vi "GCore_MFP3D_Lucy.vi"(4 "G data":dbl[](array[numeric])=[-0.02172177734863929, 0.0012861831973395592] format="%0.2f", 5 "Femto Gain (V/A)":dbl format="%#_13g", 6 "SR830 sensitivity":dbl=0.1 format="%#_6p", 7 "SR7265 sensitivity (V)":dbl=5e-07 format="%#_6p", 8 "Excitation voltage (V)":dbl format="%#_13g") -> (0 "4tR":dbl format="%#_6p", 1 "4tG":dbl format="%#_6p", 2 "2tR":dbl format="%#_6p", 3 "2tG":dbl format="%#_6p")   [LabVIEW 2019]
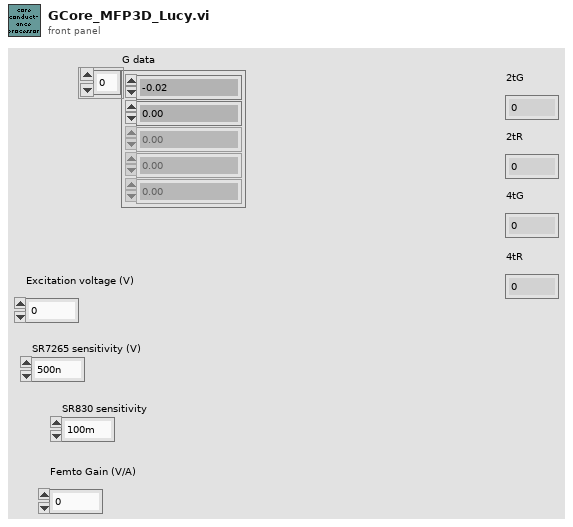
[diagram p1: front panel]
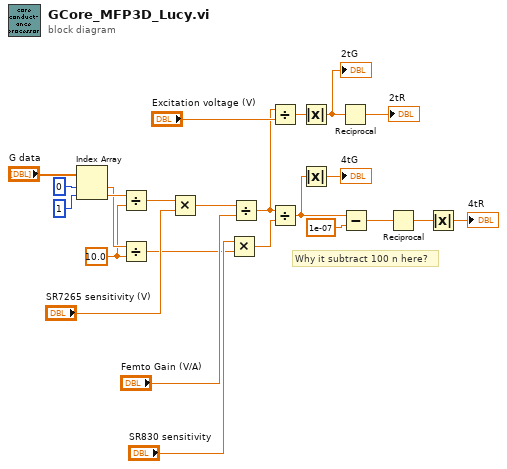
[diagram p0: block diagram]
diagram:
  w14 = 10.0 ("y")
  # "Why it subtract 100 n here?"
  n1 = Index Array(array="G data", index #1=0 ("index"), index #2=1 ("index")) -> (element #1=w15:dbl, element #2=w16:dbl)
  n2 = Divide(x=w16, y=w14) -> (x/y=w19:dbl)
  n3 = Divide(x=w15, y=w14) -> (x/y=w13:dbl)
  n4 = Multiply(x=w19, y="SR7265 sensitivity (V)") -> (x*y=w18:dbl)
  n5 = Multiply(x="SR830 sensitivity", y=w13) -> (x*y=w12:dbl)
  n6 = Divide(x=w18, y="Femto Gain (V/A)") -> (x/y=w11:dbl)
  n7 = Divide(x=w11, y="Excitation voltage (V)") -> (x/y=w10:dbl)
  n8 = Divide(x=w11, y=w12) -> (x/y=w7:dbl)
  n9 = Absolute Value(x=w10) -> (abs(x)=w9:dbl)
  "2tG" <- w9
  n10 = Absolute Value(x=w7) -> (abs(x)=→"4tG":dbl)
  n11 = Reciprocal(x=w9) -> (1/x=→"2tR":dbl)
  n12 = Subtract(x=w7, y=1e-07) -> (x-y=w5:dbl)
  n13 = Reciprocal(x=w5) -> (1/x=w4:dbl)
  n14 = Absolute Value(x=w4) -> (abs(x)=→"4tR":dbl)
